vi "PID Output Rate Limiter.vi"(7 "reinitialize? (F)":bool, 8 "dt (s)":dbl=-1.0 format="%.2f", 9 "output rate (EGU/s)":dbl=1.0 format="%.2f", 11 "input (controller output)":dbl format="%.2f") -> (0 "dt out (s)":dbl format="%.3f", 3 "output":dbl format="%.2f")   [LabVIEW 2019, in "control.lvlib"]
uses:
  control.lvlib
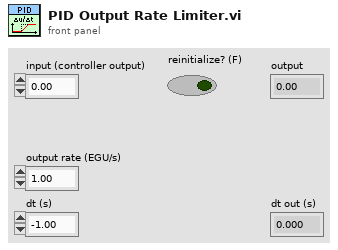
[diagram p1: front panel]
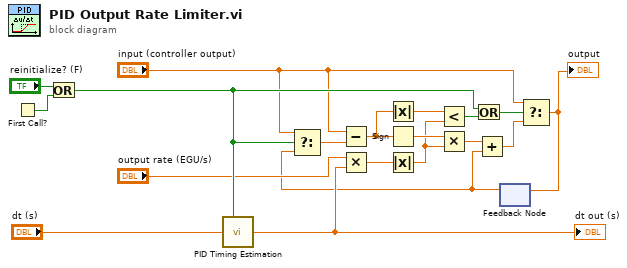
[diagram p0: block diagram]
diagram:
  n1 = First Call?() -> (First Call?: T/F=w18:bool)
  n2 = Or(x="reinitialize? (F)", y=w18) -> (x .or. y?=w17:bool)
  n3 = call "PID Timing Estimation.vi"("R"=w17, "dt (s) in"="dt (s)") -> ("dt (s) out"=w3:dbl)  [unwired: 7 in]
  "dt out (s)" <- w3
  n4 = Multiply(x="output rate (EGU/s)", y=w3) -> (x*y=w15:dbl)
  n5 = Absolute Value(x=w15) -> (abs(x)=w7:dbl)
  n6 = feedback #1() -> (w1:dbl)  [unwired: 1 in]
  n7 = Select(t="input (controller output)", s=w17, f=w1) -> (s? t:f=w10:dbl)
  n8 = Subtract(x="input (controller output)", y=w10) -> (x-y=w13:dbl)
  n9 = Absolute Value(x=w13) -> (abs(x)=w8:dbl)
  n10 = Sign(1:w13) -> (0:w11:dbl)
  n11 = Less?(x=w8, y=w7) -> (x < y?=w14:bool)
  n12 = Multiply(x=w11, y=w7) -> (x*y=w9:dbl)
  n13 = Or(x=w17, y=w14) -> (x .or. y?=w6:bool)
  n14 = Add(x=w9, y=w1) -> (x+y=w12:dbl)
  n15 = Select(t="input (controller output)", s=w6, f=w12) -> (s? t:f=w2:dbl)
  "output" <- w2
  n16 = feedback-in #1(w2) -> ()
